vi "Complex Number to String (CSG 1D Array).vi"(1 "use system decimal point (T)":bool=TRUE, 2 "precision (6)":i16, 3 "width (-)":i16, 4 "number[]":csg[](array[numeric])) -> (0 "Complex-format string []":string[](array[string]))   [LabVIEW 2018, in "Numeric Data Type.lvclass"]
doc: "<b> </b> <b> </b>\n©2013, Q Software Innovations, LLC.\n\nWritten in National Instruments LabVIEW™ 2013.\n\nAuthored by Quentin Alldredge\nQ@qsoftwareinnovations.com\nwww.qsoftwareinnovations.com\n\nAll rights reserved."
uses:
  Numeric Data Type.lvclass
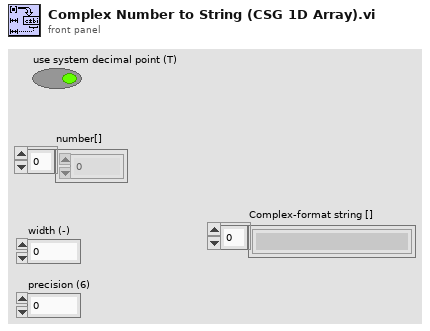
[diagram p1: front panel]
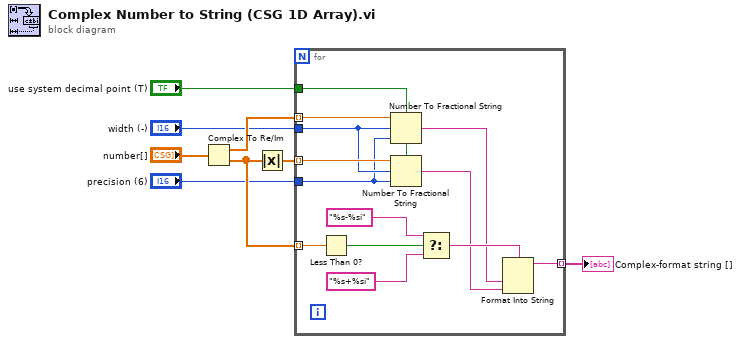
[diagram p0: block diagram]
diagram:
  n1 = Complex To Re/Im(x + iy="number[]") -> (x=w8:sgl[], y=w7:sgl[])
  n2 = Absolute Value(x=w7) -> (abs(x)=w6:sgl[])
  n3 = for {
    tunnel: w8 -> [w21] mode=indexing
    tunnel: w7 -> [w20] mode=indexing
    tunnel: w6 -> [w19] mode=indexing
    tunnel: "use system decimal point (T)" -> [w17]
    tunnel: [w11] -> w1 mode=indexing
    tunnel: "width (-)" -> [w10]
    tunnel: "precision (6)" -> [w9]
    n4 = Less Than 0?(x=w20) -> (x < 0?=w18:bool)
    n5 = Number To Fractional String(use system decimal point (T)=w17, number=w21, width (-)=w10, precision (6)=w9) -> (F-format string=w13:string)
    n6 = Number To Fractional String(use system decimal point (T)=w17, number=w19, width (-)=w10, precision (6)=w9) -> (F-format string=w12:string)
    n7 = Select(t="%s-%si", s=w18, f="%s+%si") -> (s? t:f=w14:string)
    n8 = Format Into String(format string=w14, w13, w12) -> (resulting string=w11:string)  [unwired: 2 in, 1 out]
  }
  "Complex-format string []" <- w1
